vi "Get TimeInserted.vi"(8 "error in (no error)":errorcluster, 11 "TreeNode in":refnum<class "TreeNode.lvclass">) -> (0 "error out":errorcluster, 1 "TimeInserted String out":string, 2 "timeInsertedOut":i64, 3 "TreeNode out":refnum<class "TreeNode.lvclass">)   [LabVIEW 2015, in "MDSplus.lvlib" / "TreeNode.lvclass"]
uses:
  TreeNode.lvclass
  libMDSobjectsLVShr.so
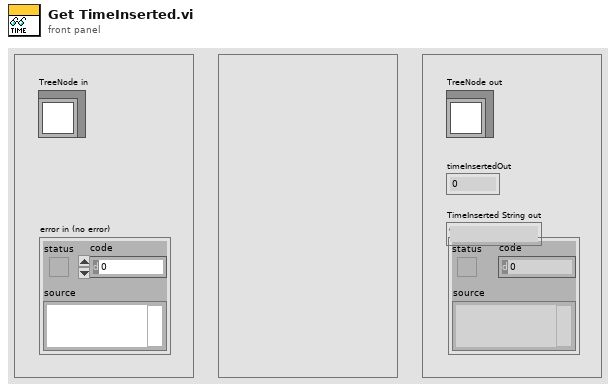
[diagram p1: front panel]
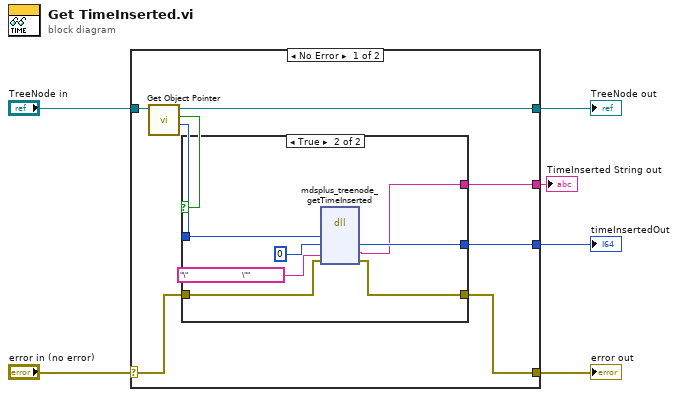
[diagram p0: block diagram]
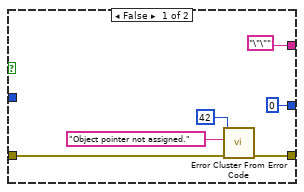
[diagram p2: hidden frame]
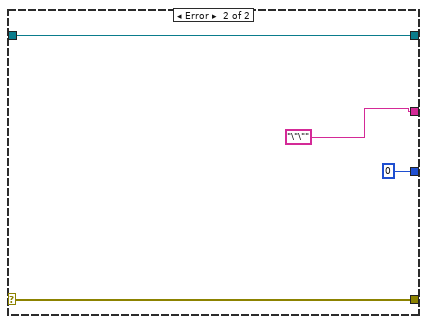
[diagram p3: hidden frame]
diagram:
  n1 = case shown="No Error" "error in (no error)" {
    selector: "error in (no error)" -> [w10 w31]
    tunnel: [w9 w31] -> w5
    tunnel: [w11 w30] -> w3
    tunnel: "TreeNode in" -> [w12 w30]
    tunnel: [w8 i64 0 ("timeInsertedOut")] -> w2
    tunnel: [w7 "\"\""] -> w1
    frame No Error {
      n2 = call-dynamic "Get Object Pointer.vi"("Data in"=w12) -> ("Object Pointer"=w13:i64, "Assigned object pointer?"=w14:bool, "Data out"=w11:refnum<class "TreeNode.lvclass">)  [unwired: 8 in]
      n3 = case shown="True" w14 {
        tunnel: w13 -> [_ w27]
        tunnel: w10 -> [w18 w26]
        tunnel: [w17 w25] -> w9
        tunnel: [i64 0 ("timeInsertedOut") w24] -> w8
        tunnel: ["\"\"" ("String value out 2") w22] -> w7
        frame False {
          n4 = call <vilib>:"Error Cluster From Error Code.vi"("error in (no error)"=w18, "error message (\"\")"="Object pointer not assigned." ("error message (\"\")"), "error code (0)"=42) -> ("error out"=w17:errorcluster)  [unwired: 6 in]
        }
        frame True {
          n5 = dll-call lib="MDSobjectsLVShr.dll" fn="mdsplus_treenode_getTimeInserted"("lvTreeNodePtr"=w27, "timeInsertedOut"=i64 0, "timeInsertedStr"="\"                           \"" ("TimeInserted String out 2"), "error"=w26) -> ("timeInsertedOut"=w24:i64, "timeInsertedStr"=w22:string, "error"=w25:errorcluster)  [unwired: 5 in, 2 out]
        }
      }
    }
    frame Error {
    }
  }
  "error out" <- w5
  "TreeNode out" <- w3
  "timeInsertedOut" <- w2
  "TimeInserted String out" <- w1
